vi "Do Core.vi"(8 "error in (no error)":errorcluster, 9 "Actor in":refnum<class "Actor.lvclass">, 11 "Reply Message":refnum<class "Save Cfg File Msg.lvclass">) -> (0 "error out":errorcluster, 1 "Actor out":refnum<class "Actor.lvclass">, 2 "Reply":variant)   [LabVIEW 2020, in "[V] Sys Cfg Base.lvlib" / "Save Cfg File Msg.lvclass"]
doc: "(<B>Filename</B>: Actor Framework.lvlib:Reply Msg.lvclass:Do Core.vi)\n\nDefines what an actor does when it receives <B>Reply Message</B>. This method also defines the <B>Reply</B> that is returned to the actor that sent <B>Reply Message</B>.\n\nBy default, this method does nothing, and <B>Reply</B> is the ancestor Message class. A child class must override this method to define behavior and specify a child of the Message class to return in the <B>Reply</B> output."
uses:
  Save Cfg File Msg.lvclass
  8396f8b9-0e62-49d3-9199-f96b831b1183.vi
  [V] Sys Cfg Base/[V] Sys Cfg Base.lvclass
  <vilib>/ActorFramework/Actor/Actor.lvclass
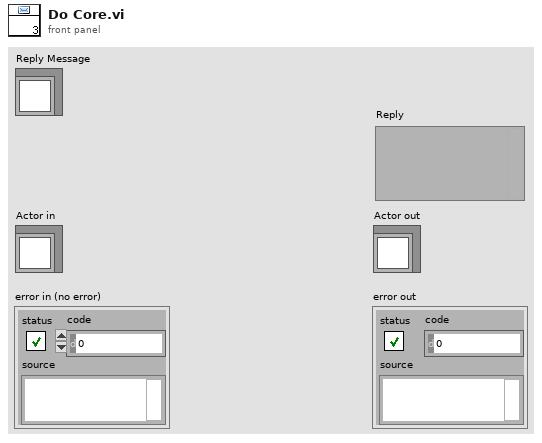
[diagram p1: front panel]
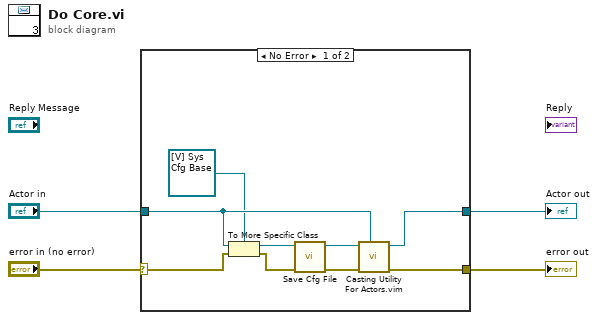
[diagram p0: block diagram]
diagram:
  n1 = case shown="No Error" "error in (no error)" {
    selector: "error in (no error)" -> [w5 w15]
    tunnel: [w9 w15] -> w3
    tunnel: [w10 w14] -> w2
    tunnel: "Actor in" -> [w12 w14]
    frame No Error {
      n2 = To More Specific Class(target class=refnum<class "[V] Sys Cfg Base.lvclass"> refnum ("Actor in"), reference=w12, error in=w5) -> (specific class reference=w13:refnum<class "[V] Sys Cfg Base.lvclass">, error out=w6:errorcluster)
      n3 = call-dynamic "Save Cfg File.vi"("error in (no error)"=w6, "[V] Sys Cfg Base in"=w13) -> ("error out"=w8:errorcluster, "[V] Sys Cfg Base out"=w11:refnum<class "[V] Sys Cfg Base.lvclass">)  [unwired: 8 in]
      n4 = call "Casting Utility For Actors.vim"("type"=w12, "error in (no error)"=w8, "Actor in"=w11) -> ("error out"=w9:errorcluster, "Actor out"=w10:refnum<class "Actor.lvclass">)  [unwired: 7 in]
    }
    frame Error {
      # "If type check fails, pass the original object out again."
    }
  }
  "error out" <- w3
  "Actor out" <- w2
